vi "Trim toque 45.vi"(6 "error in":errorcluster, 8 "MaxRead":i32, 9 "Channel in":u16) -> (0 "error out":errorcluster, 1 "Messages":T1(array[cluster]), 2 "Pass":bool, 3 "Channel out":u16)   [LabVIEW 2023]
uses:
  df35a301-8fcb-495c-91e3-c82146f18b8b.vi
  57138545-9434-49a5-ae43-5830d40555d7.vi
  2ad30504-fef7-4a6b-a16d-0a474ce5601d.vi
  Communication/PCAN2023/PCAN API.lvlib
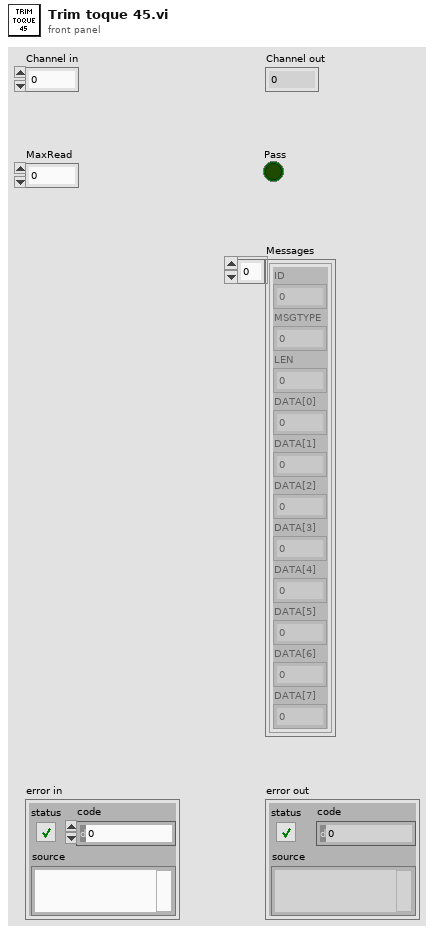
[diagram p1: front panel]
types:
  T1 = cluster{"ID":u32, "MSGTYPE":u8, "LEN":u8, "DATA[0]":u8, "DATA[1]":u8, "DATA[2]":u8, "DATA[3]":u8, "DATA[4]":u8, "DATA[5]":u8, "DATA[6]":u8, "DATA[7]":u8}[]
  T2 = cluster{"ID":u32, "MSGTYPE":u8, "LEN":u8, "DATA[0]":u8, "DATA[1]":u8, "DATA[2]":u8, "DATA[3]":u8, "DATA[4]":u8, "DATA[5]":u8, "DATA[6]":u8, "DATA[7]":u8}
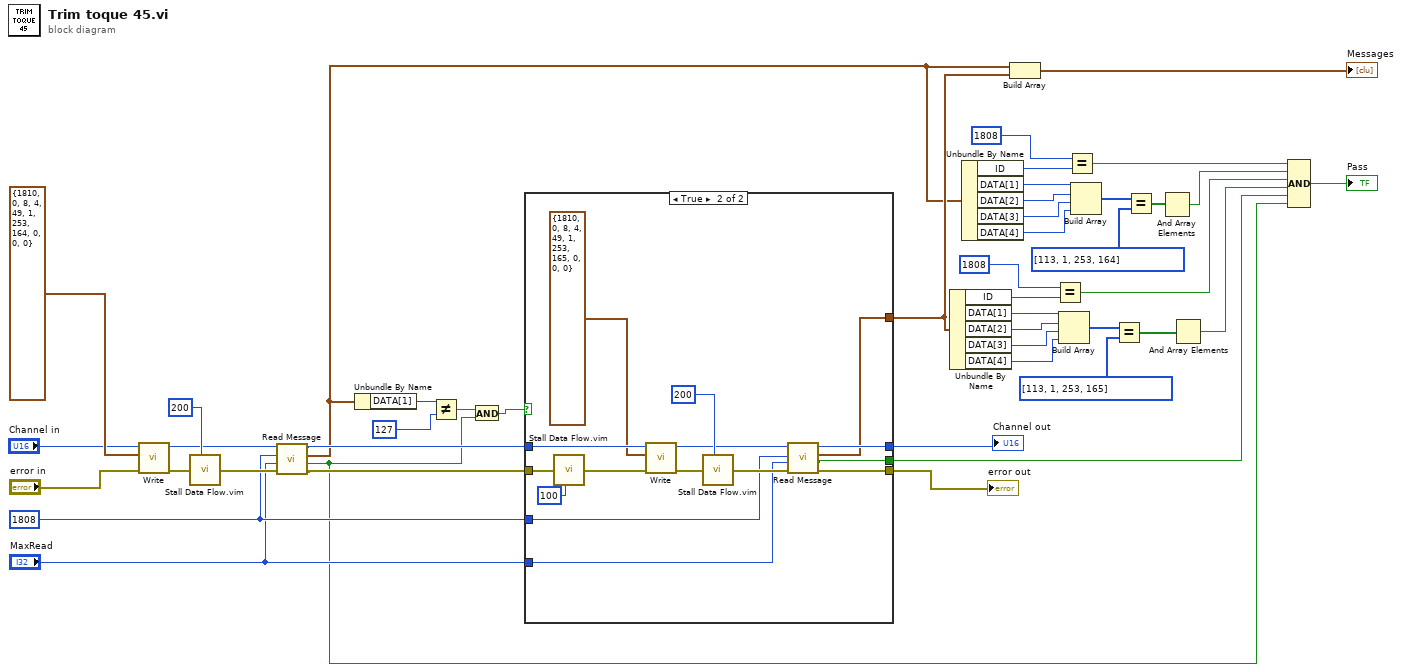
[diagram p0: block diagram]
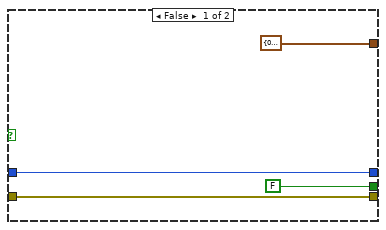
[diagram p2: hidden frame]
diagram:
  w7 = u32 1808 ("ID")
  n1 = call "Write.vi"("error in"="error in", "MessageBuffer"=T2 {"ID"=1810, "MSGTYPE"=0, "LEN"=8, "DATA[0]"=4, "DATA[1]"=49, "DATA[2]"=1, "DATA[3]"=253, "DATA[4]"=164, "DATA[5]"=0, "DATA[6]"=0, "DATA[7]"=0}, "Channel"="Channel in") -> ("error out"=w44:errorcluster, "Channel out"=w11:u16)  [unwired: 5 in, 2 out]
  n2 = call "Stall Data Flow.vim"("value in"=w44, "milliseconds to wait"=u32 200) -> ("value out"=w9:errorcluster)  [unwired: 1 out]
  n3 = call "Read Message.vi"("error in"=w9, "MaxRead"="MaxRead", "ID"=w7, "Channel in"=w11) -> ("error out"=w8:errorcluster, "Passed"=w2:bool, "Last Message"=w6:T2, "Channel out"=w10:u16)  [unwired: 3 in, 1 out]
  n4 = Unbundle By Name(w6) -> ("DATA[1]"=w12:u8)
  n5 = Not Equal?(x=w12, y=u8 127) -> (x != y?=w3:bool)
  n6 = And(x=w3, y=w2) -> (x .and. y?=w1:bool)
  n7 = case shown="True" w1 {
    tunnel: w10 -> [w48 w63]
    tunnel: w8 -> [w47 w62]
    tunnel: [w48 w56] -> w41
    tunnel: [w47 w54] -> w40
    tunnel: w7 -> [_ w53]
    tunnel: [T2 {"ID"=0, "MSGTYPE"=0, "LEN"=0, "DATA[0]"=0, "DATA[1]"=0, "DATA[2]"=0, "DATA[3]"=0, "DATA[4]"=0, "DATA[5]"=0, "DATA[6]"=0, "DATA[7]"=0} ("MessageBuffer out") w51] -> w15
    tunnel: "MaxRead" -> [_ w52]
    tunnel: [FALSE ("Passed") w50] -> w4
    frame False {
    }
    frame True {
      n8 = call "Stall Data Flow.vim"("value in"=w62, "milliseconds to wait"=u32 100) -> ("value out"=w60:errorcluster)  [unwired: 1 out]
      n9 = call "Write.vi"("error in"=w60, "MessageBuffer"=T2 {"ID"=1810, "MSGTYPE"=0, "LEN"=8, "DATA[0]"=4, "DATA[1]"=49, "DATA[2]"=1, "DATA[3]"=253, "DATA[4]"=165, "DATA[5]"=0, "DATA[6]"=0, "DATA[7]"=0}, "Channel"=w63) -> ("error out"=w64:errorcluster, "Channel out"=w57:u16)  [unwired: 5 in, 2 out]
      n10 = call "Stall Data Flow.vim"("value in"=w64, "milliseconds to wait"=u32 200) -> ("value out"=w55:errorcluster)  [unwired: 1 out]
      n11 = call "Read Message.vi"("error in"=w55, "MaxRead"=w52, "ID"=w53, "Channel in"=w57) -> ("error out"=w54:errorcluster, "Passed"=w50:bool, "Last Message"=w51:T2, "Channel out"=w56:u16)  [unwired: 3 in, 1 out]
    }
  }
  "error out" <- w40
  "Channel out" <- w41
  n12 = Unbundle By Name(w15) -> ("ID"=w26:u32, "DATA[1]"=w22:u8, "DATA[2]"=w23:u8, "DATA[3]"=w24:u8, "DATA[4]"=w25:u8)
  n13 = Unbundle By Name(w6) -> ("ID"=w34:u32, "DATA[1]"=w38:u8, "DATA[2]"=w37:u8, "DATA[3]"=w36:u8, "DATA[4]"=w35:u8)
  n14 = Build Array(w6, w15) -> (→"Messages":T1)
  n15 = Equal?(x=u32 1808, y=w26) -> (x = y?=w21:bool)
  n16 = Build Array(w22, w23, w24, w25) -> (w28:u8[])
  n17 = Equal?(x=u32 1808, y=w34) -> (x = y?=w30:bool)
  n18 = Build Array(w38, w37, w36, w35) -> (w32:u8[])
  n19 = Equal?(x=w28, y=u8[] [113, 1, 253, 165]) -> (x = y?=w19:bool[])
  n20 = Equal?(x=w32, y=u8[] [113, 1, 253, 164]) -> (x = y?=w20:bool[])
  n21 = And Array Elements(Boolean array=w20) -> (logical AND=w18:bool)
  n22 = And Array Elements(Boolean array=w19) -> (logical AND=w17:bool)
  n23 = Compound Arithmetic op=AND(w30, w18, w21, w17, w4, w2) -> (→"Pass":bool)
